vi "UnloadAction.vi"(8 "error in (no error)":errorcluster caption="entrée d'erreur (pas d'erreur)", 11 "Tools In":refnum<class "AppliedMotionDrive.lvclass"> caption="DNL_LabVIEW Object in") -> (0 "error out":errorcluster caption="sortie d'erreur", 3 "Tools Out":refnum<class "AppliedMotionDrive.lvclass"> caption="DNL_LabVIEW Object out")   [LabVIEW 2019, in "AppliedMotionDrive.lvclass"]
uses:
  AppliedMotionDrive.lvclass
  C:/Programmes Labview/LabscanV1A/DevicesClass/BaseDevice/BaseDevice.lvclass
  BaseDevice/BaseDevice.lvclass
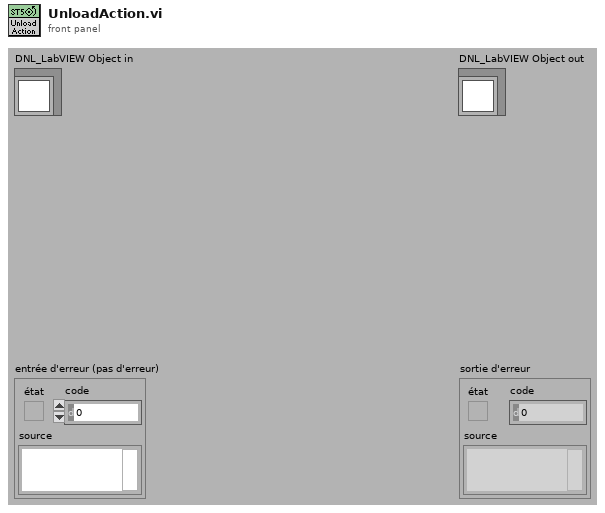
[diagram p1: front panel]
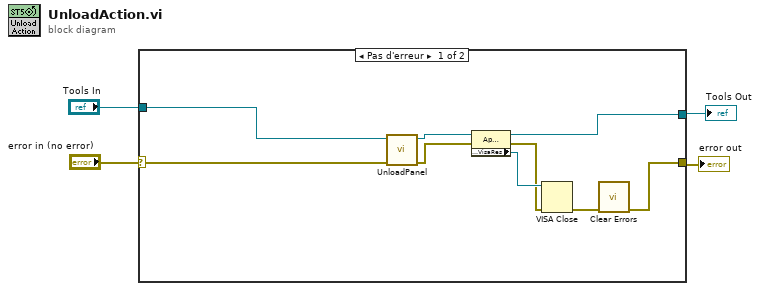
[diagram p0: block diagram]
diagram:
  n1 = case shown="Pas d'erreur" "error in (no error)" {
    selector: "error in (no error)" -> [w13 w14]
    tunnel: [w5 w14] -> w3
    tunnel: [w6 w15] -> w2
    tunnel: "Tools In" -> [w12 w15]
    frame No Error {
      n2 = call "UnloadPanel.vi"("error in (no error)"=w13, "Device en entrée"=w12) -> ("error out"=w7:errorcluster, "Device en sortie"=w11:refnum<class "AppliedMotionDrive.lvclass">)  [unwired: 8 in]
      n3 = property class="AppliedMotionDrive.lvclass"(reference=w11, error in=w7) -> (reference out=w6:refnum<class "AppliedMotionDrive.lvclass">, error out=w9:errorcluster, "Accessor:VisaRes"=w10:refnum<visa-resource-name>)
      n4 = VISA Close(VISA resource name=w10, error in (no error)=w9) -> (error out=w8:errorcluster)
      n5 = call <vilib>:"Clear Errors.vi"("error in (no error)"=w8) -> ("error out"=w5:errorcluster)  [unwired: 5 in, 1 out]
    }
    frame Error {
    }
  }
  "error out" <- w3
  "Tools Out" <- w2
